vi "Is Valid Path.vi"(9 "max dist":dbl, 10 "Waypoints":cluster{"x":dbl, "y":dbl, "th":dbl}[](array[cluster]), 11 "ball pts":cluster{"x":dbl, "y":dbl, "th":dbl}[](array[cluster])) -> (3 "is valid?":bool)   [LabVIEW 2019]
panel:
  out "max dist out":dbl
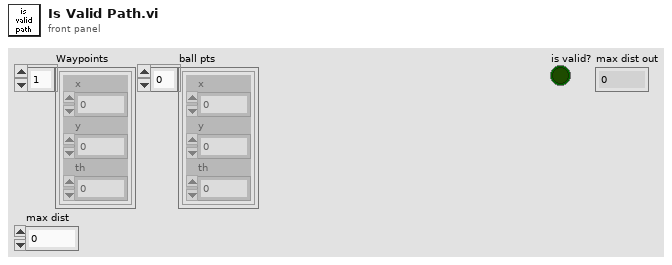
[diagram p1: front panel]
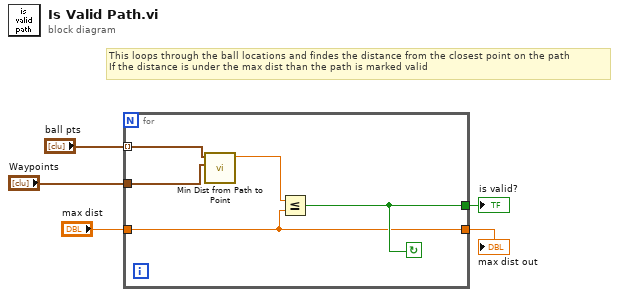
[diagram p0: block diagram]
diagram:
  # "This loops through the ball locations and findes the distance from the closest point on the path\nIf the distance is under the max dist than the path is marked valid"
  n1 = for {
    tunnel: "Waypoints" -> [w10]
    tunnel: "ball pts" -> [w9] mode=indexing
    tunnel: "max dist" -> [w6]
    tunnel: [w7] -> w2
    tunnel: [w6] -> w1
    stop <- w7 continue-if-true
    n2 = call "Min Dist from Path to Point.vi"("point"=w9, "Waypoints"=w10) -> ("min dist"=w8:dbl)  [unwired: 8 in]
    n3 = Less Or Equal?(x=w8, y=w6) -> (x <= y?=w7:bool)
  }
  "is valid?" <- w2
  "max dist out" <- w1
